vi "ZK_Main.vi"() -> ()   [LabVIEW 2018]
uses:
  C:/Users/rshang/Desktop/2020_APZK_LV360_Ricky/LabVIEWZOOKEPPER_V3/ClassLibrary_ZK.dll
  2020_APZK_LV360_Ricky/LabVIEWZOOKEPPER_V3/ClassLibrary_ZK.dll
  <vilib>/Utility/inputDevices.llb/keyboardAcquire.vi
  <vilib>/Utility/inputDevices.llb/closeKeyboard.vi
panel:
  out "Found?":bool=TRUE
  in  "Auto\n(Press keyboad\n A to stop)":bool
  in  "exe position":T1={"LU"={"x"=1456.0, "y"=98.0}, " RD"={"x"=1806.0, "y"=511.0}}
  out "Array":dbl[][](array[numeric])=[[0.0, 7.0, 4.0, 1.0, 7.0, 1.0, 7.0, 1.0], [5.0, 4.0, 6.0, 3.0, 7.0, 7.0, 1.0, 4.0], [3.0, 2.0, 4.0, 6.0, 1.0, 2.0, 7.0, 4.0], [5.0, 2.0, 6.0, 5.0, 4.0, 1.0, 4.0, 6.0], [3.0, 1.0, 2.0, 6.0, 5.0, 2.0, 4.0, 3.0], [4.0, 5.0, 1.0, 6.0, 1.0, 1.0, 7.0, 3.0], [6.0, 1.0, 2.0, 4.0, 4.0, 7.0, 3.0, 1.0], [6.0, 5.0, 2.0, 7.0, 3.0, 5.0, 3.0, 1.0]]
  out "Title":string="Zookeeper LabVIEW auto-player"
  out "Auto":bool
  in  "mouse setting":cluster{"X1":i32, "Y1":i32, "X2":i32, "Y2":i32}={"X1"=1479, "Y1"=217, "X2"=1733, "Y2"=457}
  in  "stop":bool
  out "Calibrated Matches 2":T2(array[cluster])=[[{"Position"={"x"=75.00092, "y"=255.0092}, "Angle"=0.0, "Scale"=1.0, "Score"=933.23773, "Bounding Box"=[{"x"=58.000923, "y"=238.0092}, {"x"=91.00092, "y"=238.0092}, {"x"=91.00092, "y"=271.00922}, {"x"=58.000923, "y"=271.00922}, {"x"=58.000923, "y"=238.0092}]}, {"Position"={"x"=279.0, "y"=323.0}, "Angle"=0.0, "Scale"=1.0, "Score"=932.08344, "Bounding Box"=[{"x"=262.0, "y"=306.0}, {"x"=295.0, "y"=306.0}, {"x"=295.0, "y"=339.0}, {"x"=262.0, "y"=339.0}, {"x"=262.0, "y"=306.0}]}, {"Position"={"x"=210.99873, "y"=119.0105}, "Angle"=0.0, "Scale"=1.0, "Score"=930.9997, "Bounding Box"=[{"x"=193.99873, "y"=102.0105}, {"x"=226.99873, "y"=102.0105}, {"x"=226.99873, "y"=135.0105}, {"x"=193.99873, "y"=135.0105}, {"x"=193.99873, "y"=102.0105}]}, {"Position"={"x"=176.99084, "y"=289.02286}, "Angle"=0.0, "Scale"=1.0, "Score"=925.0761, "Bounding Box"=[{"x"=159.99084, "y"=272.02286}, {"x"=192.99084, "y"=272.02286}, {"x"=192.99084, "y"=305.02286}, {"x"=159.99084, "y"=305.02286}, {"x"=159.99084, "y"=272.02286}]}, {"Position"={"x"=210.99141, "y"=288.9893}, "Angle"=0.0, "Scale"=1.0, "Score"=925.0041, "Bounding Box"=[{"x"=193.99141, "y"=271.9893}, {"x"=226.99141, "y"=271.9893}, {"x"=226.99141, "y"=304.9893}, {"x"=193.99141, "y"=304.9893}, {"x"=193.99141, "y"=271.9893}]}, {"Position"={"x"=142.99681, "y"=119.04378}, "Angle"=0.0, "Scale"=1.0, "Score"=920.4134, "Bounding Box"=[{"x"=125.99681, "y"=102.04378}, {"x"=158.99681, "y"=102.04378}, {"x"=158.99681, "y"=135.04378}, {"x"=125.99681, "y"=135.04378}, {"x"=125.99681, "y"=102.04378}]}, {"Position"={"x"=278.99835, "y"=119.04145}, "Angle"=0.0, "Scale"=1.0, "Score"=912.4555, "Bounding Box"=[{"x"=261.99835, "y"=102.04145}, {"x"=294.99835, "y"=102.04145}, {"x"=294.99835, "y"=135.04144}, {"x"=261.99835, "y"=135.04144}, {"x"=261.99835, "y"=102.04145}]}, {"Position"={"x"=245.00299, "y"=153.00949}, "Angle"=0.0, "Scale"=1.0, "Score"=905.00775, "Bounding Box"=[{"x"=228.00299, "y"=136.00949}, {"x"=261.003, "y"=136.00949}, {"x"=261.003, "y"=169.00949}, {"x"=228.00299, "y"=169.00949}, {"x"=228.00299, "y"=136.00949}]}, {"Position"={"x"=177.00247, "y"=186.99414}, "Angle"=0.0, "Scale"=1.0, "Score"=904.1407, "Bounding Box"=[{"x"=160.00247, "y"=169.99414}, {"x"=193.00247, "y"=169.99414}, {"x"=193.00247, "y"=202.99414}, {"x"=160.00247, "y"=202.99414}, {"x"=160.00247, "y"=169.99414}]}, {"Position"={"x"=210.99931, "y"=220.98695}, "Angle"=0.0, "Scale"=1.0, "Score"=901.1566, "Bounding Box"=[{"x"=193.99931, "y"=203.98695}, {"x"=226.99931, "y"=203.98695}, {"x"=226.99931, "y"=236.98695}, {"x"=193.99931, "y"=236.98695}, {"x"=193.99931, "y"=203.98695}]}, {"Position"={"x"=109.00134, "y"=289.00165}, "Angle"=0.0, "Scale"=1.0, "Score"=887.957, "Bounding Box"=[{"x"=92.00134, "y"=272.00165}, {"x"=125.00134, "y"=272.00165}, {"x"=125.00134, "y"=305.00165}, {"x"=92.00134, "y"=305.00165}, {"x"=92.00134, "y"=272.00165}]}, {"Position"={"x"=75.00068, "y"=323.03723}, "Angle"=0.0, "Scale"=1.0, "Score"=884.5231, "Bounding Box"=[{"x"=58.00068, "y"=306.03723}, {"x"=91.00068, "y"=306.03723}, {"x"=91.00068, "y"=339.03723}, {"x"=58.00068, "y"=339.03723}, {"x"=58.00068, "y"=306.03723}]}, {"Position"={"x"=273.11758, "y"=362.57874}, "Angle"=0.0, "Scale"=1.0, "Score"=841.5791, "Bounding Box"=[{"x"=256.11758, "y"=345.57874}, {"x"=289.11758, "y"=345.57874}, {"x"=289.11758, "y"=378.57874}, {"x"=256.11758, "y"=378.57874}, {"x"=256.11758, "y"=345.57874}]}], [{"Position"={"x"=107.986984, "y"=323.99716}, "Angle"=0.0, "Scale"=1.0, "Score"=931.8045, "Bounding Box"=[{"x"=92.986984, "y"=307.99716}, {"x"=121.986984, "y"=307.99716}, {"x"=121.986984, "y"=338.99716}, {"x"=92.986984, "y"=338.99716}, {"x"=92.986984, "y"=307.99716}]}, {"Position"={"x"=74.068016, "y"=221.99124}, "Angle"=0.0, "Scale"=1.0, "Score"=925.1344, "Bounding Box"=[{"x"=59.068016, "y"=205.99124}, {"x"=88.068016, "y"=205.99124}, {"x"=88.068016, "y"=236.99124}, {"x"=59.068016, "y"=236.99124}, {"x"=59.068016, "y"=205.99124}]}, {"Position"={"x"=210.09818, "y"=256.00165}, "Angle"=0.0, "Scale"=1.0, "Score"=920.25055, "Bounding Box"=[{"x"=195.09818, "y"=240.00165}, {"x"=224.09818, "y"=240.00165}, {"x"=224.09818, "y"=271.00165}, {"x"=195.09818, "y"=271.00165}, {"x"=195.09818, "y"=240.00165}]}, {"Position"={"x"=108.11167, "y"=256.0057}, "Angle"=0.0, "Scale"=1.0, "Score"=915.52545, "Bounding Box"=[{"x"=93.11167, "y"=240.0057}, {"x"=122.11167, "y"=240.0057}, {"x"=122.11167, "y"=271.0057}, {"x"=93.11167, "y"=271.0057}, {"x"=93.11167, "y"=240.0057}]}, {"Position"={"x"=209.99649, "y"=188.00977}, "Angle"=0.0, "Scale"=1.0, "Score"=910.0421, "Bounding Box"=[{"x"=194.99649, "y"=172.00977}, {"x"=223.99649, "y"=172.00977}, {"x"=223.99649, "y"=203.00977}, {"x"=194.99649, "y"=203.00977}, {"x"=194.99649, "y"=172.00977}]}, {"Position"={"x"=107.98176, "y"=357.98648}, "Angle"=0.0, "Scale"=1.0, "Score"=894.9287, "Bounding Box"=[{"x"=92.98176, "y"=341.98648}, {"x"=121.98176, "y"=341.98648}, {"x"=121.98176, "y"=372.98648}, {"x"=92.98176, "y"=372.98648}, {"x"=92.98176, "y"=341.98648}]}, {"Position"={"x"=74.02244, "y"=188.00812}, "Angle"=0.0, "Scale"=1.0, "Score"=888.29694, "Bounding Box"=[{"x"=59.022438, "y"=172.00812}, {"x"=88.02244, "y"=172.00812}, {"x"=88.02244, "y"=203.00812}, {"x"=59.022438, "y"=203.00812}, {"x"=59.022438, "y"=172.00812}]}, {"Position"={"x"=0.0, "y"=0.0}, "Angle"=0.0, "Scale"=0.0, "Score"=0.0, "Bounding Box"=[]}, {"Position"={"x"=0.0, "y"=0.0}, "Angle"=0.0, "Scale"=0.0, "Score"=0.0, "Bounding Box"=[]}, {"Position"={"x"=0.0, "y"=0.0}, "Angle"=0.0, "Scale"=0.0, "Score"=0.0, "Bounding Box"=[]}, {"Position"={"x"=0.0, "y"=0.0}, "Angle"=0.0, "Scale"=0.0, "Score"=0.0, "Bounding Box"=[]}, {"Position"={"x"=0.0, "y"=0.0}, "Angle"=0.0, "Scale"=0.0, "Score"=0.0, "Bounding Box"=[]}, {"Position"={"x"=0.0, "y"=0.0}, "Angle"=0.0, "Scale"=0.0, "Score"=0.0, "Bounding Box"=[]}], [{"Position"={"x"=277.90146, "y"=289.0273}, "Angle"=0.0, "Scale"=1.0, "Score"=926.91986, "Bounding Box"=[{"x"=261.90146, "y"=272.0273}, {"x"=292.90146, "y"=272.0273}, {"x"=292.90146, "y"=305.0273}, {"x"=261.90146, "y"=305.0273}, {"x"=261.90146, "y"=272.0273}]}, {"Position"={"x"=142.0333, "y"=153.05386}, "Angle"=0.0, "Scale"=1.0, "Score"=920.6298, "Bounding Box"=[{"x"=126.033295, "y"=136.05386}, {"x"=157.0333, "y"=136.05386}, {"x"=157.0333, "y"=169.05386}, {"x"=126.033295, "y"=169.05386}, {"x"=126.033295, "y"=136.05386}]}, {"Position"={"x"=176.00894, "y"=357.03848}, "Angle"=0.0, "Scale"=1.0, "Score"=920.4684, "Bounding Box"=[{"x"=160.00894, "y"=340.03848}, {"x"=191.00894, "y"=340.03848}, {"x"=191.00894, "y"=373.03848}, {"x"=160.00894, "y"=373.03848}, {"x"=160.00894, "y"=340.03848}]}, {"Position"={"x"=243.82567, "y"=357.03494}, "Angle"=0.0, "Scale"=1.0, "Score"=917.59546, "Bounding Box"=[{"x"=227.82567, "y"=340.03494}, {"x"=258.82568, "y"=340.03494}, {"x"=258.82568, "y"=373.03494}, {"x"=227.82567, "y"=373.03494}, {"x"=227.82567, "y"=340.03494}]}, {"Position"={"x"=40.012535, "y"=187.0207}, "Angle"=0.0, "Scale"=1.0, "Score"=903.5547, "Bounding Box"=[{"x"=24.012535, "y"=170.0207}, {"x"=55.012535, "y"=170.0207}, {"x"=55.012535, "y"=203.0207}, {"x"=24.012535, "y"=203.0207}, {"x"=24.012535, "y"=170.0207}]}, {"Position"={"x"=40.08889, "y"=255.02586}, "Angle"=0.0, "Scale"=1.0, "Score"=899.9424, "Bounding Box"=[{"x"=24.08889, "y"=238.02586}, {"x"=55.08889, "y"=238.02586}, {"x"=55.08889, "y"=271.02588}, {"x"=24.08889, "y"=271.02588}, {"x"=24.08889, "y"=238.02586}]}, {"Position"={"x"=244.2408, "y"=323.06232}, "Angle"=0.0, "Scale"=1.0, "Score"=899.3051, "Bounding Box"=[{"x"=228.2408, "y"=306.06232}, {"x"=259.24078, "y"=306.06232}, {"x"=259.24078, "y"=339.06232}, {"x"=228.2408, "y"=339.06232}, {"x"=228.2408, "y"=306.06232}]}, {"Position"={"x"=277.75967, "y"=255.03061}, "Angle"=0.0, "Scale"=1.0, "Score"=894.2649, "Bounding Box"=[{"x"=261.75967, "y"=238.03061}, {"x"=292.75967, "y"=238.03061}, {"x"=292.75967, "y"=271.0306}, {"x"=261.75967, "y"=271.0306}, {"x"=261.75967, "y"=238.03061}]}, {"Position"={"x"=0.0, "y"=0.0}, "Angle"=0.0, "Scale"=0.0, "Score"=0.0, "Bounding Box"=[]}, {"Position"={"x"=0.0, "y"=0.0}, "Angle"=0.0, "Scale"=0.0, "Score"=0.0, "Bounding Box"=[]}, {"Position"={"x"=0.0, "y"=0.0}, "Angle"=0.0, "Scale"=0.0, "Score"=0.0, "Bounding Box"=[]}, {"Position"={"x"=0.0, "y"=0.0}, "Angle"=0.0, "Scale"=0.0, "Score"=0.0, "Bounding Box"=[]}, {"Position"={"x"=0.0, "y"=0.0}, "Angle"=0.0, "Scale"=0.0, "Score"=0.0, "Bounding Box"=[]}], [{"Position"={"x"=245.00069, "y"=254.18097}, "Angle"=0.0, "Scale"=1.0, "Score"=954.2915, "Bounding Box"=[{"x"=230.00069, "y"=238.18097}, {"x"=260.00067, "y"=238.18097}, {"x"=260.00067, "y"=269.18097}, {"x"=230.00069, "y"=269.18097}, {"x"=230.00069, "y"=238.18097}]}, {"Position"={"x"=279.13513, "y"=152.48029}, "Angle"=0.0, "Scale"=1.0, "Score"=940.6921, "Bounding Box"=[{"x"=264.13513, "y"=136.48029}, {"x"=294.13513, "y"=136.48029}, {"x"=294.13513, "y"=167.48029}, {"x"=264.13513, "y"=167.48029}, {"x"=264.13513, "y"=136.48029}]}, {"Position"={"x"=109.067566, "y"=186.16963}, "Angle"=0.0, "Scale"=1.0, "Score"=938.7648, "Bounding Box"=[{"x"=94.067566, "y"=170.16963}, {"x"=124.067566, "y"=170.16963}, {"x"=124.067566, "y"=201.16963}, {"x"=94.067566, "y"=201.16963}, {"x"=94.067566, "y"=170.16963}]}, {"Position"={"x"=177.16257, "y"=322.33588}, "Angle"=0.0, "Scale"=1.0, "Score"=933.9336, "Bounding Box"=[{"x"=162.16257, "y"=306.33588}, {"x"=192.16257, "y"=306.33588}, {"x"=192.16257, "y"=337.33588}, {"x"=162.16257, "y"=337.33588}, {"x"=162.16257, "y"=306.33588}]}, {"Position"={"x"=75.14856, "y"=152.44539}, "Angle"=0.0, "Scale"=1.0, "Score"=927.445, "Bounding Box"=[{"x"=60.14856, "y"=136.44539}, {"x"=90.14856, "y"=136.44539}, {"x"=90.14856, "y"=167.44539}, {"x"=60.14856, "y"=167.44539}, {"x"=60.14856, "y"=136.44539}]}, {"Position"={"x"=108.93101, "y"=118.46414}, "Angle"=0.0, "Scale"=1.0, "Score"=922.298, "Bounding Box"=[{"x"=93.93101, "y"=102.46414}, {"x"=123.93101, "y"=102.46414}, {"x"=123.93101, "y"=133.46414}, {"x"=93.93101, "y"=133.46414}, {"x"=93.93101, "y"=102.46414}]}, {"Position"={"x"=143.0, "y"=323.0}, "Angle"=0.0, "Scale"=1.0, "Score"=915.732, "Bounding Box"=[{"x"=128.0, "y"=307.0}, {"x"=158.0, "y"=307.0}, {"x"=158.0, "y"=338.0}, {"x"=128.0, "y"=338.0}, {"x"=128.0, "y"=307.0}]}, {"Position"={"x"=41.060474, "y"=288.27094}, "Angle"=0.0, "Scale"=1.0, "Score"=914.88336, "Bounding Box"=[{"x"=26.060474, "y"=272.27094}, {"x"=56.060474, "y"=272.27094}, {"x"=56.060474, "y"=303.27094}, {"x"=26.060474, "y"=303.27094}, {"x"=26.060474, "y"=272.27094}]}, {"Position"={"x"=244.9803, "y"=220.15024}, "Angle"=0.0, "Scale"=1.0, "Score"=913.309, "Bounding Box"=[{"x"=229.9803, "y"=204.15024}, {"x"=259.9803, "y"=204.15024}, {"x"=259.9803, "y"=235.15024}, {"x"=229.9803, "y"=235.15024}, {"x"=229.9803, "y"=204.15024}]}, {"Position"={"x"=279.1057, "y"=185.95796}, "Angle"=0.0, "Scale"=1.0, "Score"=905.5621, "Bounding Box"=[{"x"=264.1057, "y"=169.95796}, {"x"=294.1057, "y"=169.95796}, {"x"=294.1057, "y"=200.95796}, {"x"=264.1057, "y"=200.95796}, {"x"=264.1057, "y"=169.95796}]}, {"Position"={"x"=176.76869, "y"=220.71819}, "Angle"=0.0, "Scale"=1.0, "Score"=901.4693, "Bounding Box"=[{"x"=161.76869, "y"=204.71819}, {"x"=191.76869, "y"=204.71819}, {"x"=191.76869, "y"=235.71819}, {"x"=161.76869, "y"=235.71819}, {"x"=161.76869, "y"=204.71819}]}, {"Position"={"x"=0.0, "y"=0.0}, "Angle"=0.0, "Scale"=0.0, "Score"=0.0, "Bounding Box"=[]}, {"Position"={"x"=0.0, "y"=0.0}, "Angle"=0.0, "Scale"=0.0, "Score"=0.0, "Bounding Box"=[]}], [{"Position"={"x"=74.0, "y"=355.0}, "Angle"=0.0, "Scale"=1.0, "Score"=919.12885, "Bounding Box"=[{"x"=58.0, "y"=339.0}, {"x"=90.0, "y"=339.0}, {"x"=90.0, "y"=371.0}, {"x"=58.0, "y"=371.0}, {"x"=58.0, "y"=339.0}]}, {"Position"={"x"=73.991066, "y"=287.9914}, "Angle"=0.0, "Scale"=1.0, "Score"=878.5044, "Bounding Box"=[{"x"=57.991066, "y"=271.9914}, {"x"=89.991066, "y"=271.9914}, {"x"=89.991066, "y"=303.9914}, {"x"=57.991066, "y"=303.9914}, {"x"=57.991066, "y"=271.9914}]}, {"Position"={"x"=27.626839, "y"=210.72752}, "Angle"=0.0, "Scale"=1.0, "Score"=863.36957, "Bounding Box"=[{"x"=11.626839, "y"=194.72752}, {"x"=43.62684, "y"=194.72752}, {"x"=43.62684, "y"=226.72752}, {"x"=11.626839, "y"=226.72752}, {"x"=11.626839, "y"=194.72752}]}, {"Position"={"x"=209.92537, "y"=356.0048}, "Angle"=0.0, "Scale"=1.0, "Score"=856.84375, "Bounding Box"=[{"x"=193.92537, "y"=340.0048}, {"x"=225.92537, "y"=340.0048}, {"x"=225.92537, "y"=372.0048}, {"x"=193.92537, "y"=372.0048}, {"x"=193.92537, "y"=340.0048}]}, {"Position"={"x"=175.98193, "y"=253.99306}, "Angle"=0.0, "Scale"=1.0, "Score"=848.5472, "Bounding Box"=[{"x"=159.98193, "y"=237.99306}, {"x"=191.98193, "y"=237.99306}, {"x"=191.98193, "y"=269.99304}, {"x"=159.98193, "y"=269.99304}, {"x"=159.98193, "y"=237.99306}]}, {"Position"={"x"=141.95236, "y"=220.00485}, "Angle"=0.0, "Scale"=1.0, "Score"=844.96405, "Bounding Box"=[{"x"=125.95236, "y"=204.00485}, {"x"=157.95236, "y"=204.00485}, {"x"=157.95236, "y"=236.00485}, {"x"=125.95236, "y"=236.00485}, {"x"=125.95236, "y"=204.00485}]}, {"Position"={"x"=27.773817, "y"=140.42613}, "Angle"=0.0, "Scale"=1.0, "Score"=830.67377, "Bounding Box"=[{"x"=11.773817, "y"=124.42613}, {"x"=43.77382, "y"=124.42613}, {"x"=43.77382, "y"=156.42613}, {"x"=11.773817, "y"=156.42613}, {"x"=11.773817, "y"=124.42613}]}, {"Position"={"x"=191.0, "y"=374.0}, "Angle"=0.0, "Scale"=1.0, "Score"=814.83405, "Bounding Box"=[{"x"=175.0, "y"=358.0}, {"x"=207.0, "y"=358.0}, {"x"=207.0, "y"=390.0}, {"x"=175.0, "y"=390.0}, {"x"=175.0, "y"=358.0}]}, {"Position"={"x"=0.0, "y"=0.0}, "Angle"=0.0, "Scale"=0.0, "Score"=0.0, "Bounding Box"=[]}, {"Position"={"x"=0.0, "y"=0.0}, "Angle"=0.0, "Scale"=0.0, "Score"=0.0, "Bounding Box"=[]}, {"Position"={"x"=0.0, "y"=0.0}, "Angle"=0.0, "Scale"=0.0, "Score"=0.0, "Bounding Box"=[]}, {"Position"={"x"=0.0, "y"=0.0}, "Angle"=0.0, "Scale"=0.0, "Score"=0.0, "Bounding Box"=[]}, {"Position"={"x"=0.0, "y"=0.0}, "Angle"=0.0, "Scale"=0.0, "Score"=0.0, "Bounding Box"=[]}], [{"Position"={"x"=108.99241, "y"=153.01335}, "Angle"=0.0, "Scale"=1.0, "Score"=950.8153, "Bounding Box"=[{"x"=92.99241, "y"=136.01335}, {"x"=123.99241, "y"=136.01335}, {"x"=123.99241, "y"=170.01335}, {"x"=92.99241, "y"=170.01335}, {"x"=92.99241, "y"=136.01335}]}, {"Position"={"x"=109.00232, "y"=221.00328}, "Angle"=0.0, "Scale"=1.0, "Score"=950.37427, "Bounding Box"=[{"x"=93.00232, "y"=204.00328}, {"x"=124.00232, "y"=204.00328}, {"x"=124.00232, "y"=238.00328}, {"x"=93.00232, "y"=238.00328}, {"x"=93.00232, "y"=204.00328}]}, {"Position"={"x"=142.97572, "y"=187.00519}, "Angle"=0.0, "Scale"=1.0, "Score"=949.1306, "Bounding Box"=[{"x"=126.97572, "y"=170.00519}, {"x"=157.97572, "y"=170.00519}, {"x"=157.97572, "y"=204.00519}, {"x"=126.97572, "y"=204.00519}, {"x"=126.97572, "y"=170.00519}]}, {"Position"={"x"=278.84097, "y"=220.9837}, "Angle"=0.0, "Scale"=1.0, "Score"=935.6025, "Bounding Box"=[{"x"=262.84097, "y"=203.9837}, {"x"=293.84097, "y"=203.9837}, {"x"=293.84097, "y"=237.9837}, {"x"=262.84097, "y"=237.9837}, {"x"=262.84097, "y"=203.9837}]}, {"Position"={"x"=143.0, "y"=289.0}, "Angle"=0.0, "Scale"=1.0, "Score"=926.99817, "Bounding Box"=[{"x"=127.0, "y"=272.0}, {"x"=158.0, "y"=272.0}, {"x"=158.0, "y"=306.0}, {"x"=127.0, "y"=306.0}, {"x"=127.0, "y"=272.0}]}, {"Position"={"x"=142.79024, "y"=255.01186}, "Angle"=0.0, "Scale"=1.0, "Score"=919.38403, "Bounding Box"=[{"x"=126.79024, "y"=238.01186}, {"x"=157.79024, "y"=238.01186}, {"x"=157.79024, "y"=272.01184}, {"x"=126.79024, "y"=272.01184}, {"x"=126.79024, "y"=238.01186}]}, {"Position"={"x"=41.008556, "y"=323.00058}, "Angle"=0.0, "Scale"=1.0, "Score"=916.4105, "Bounding Box"=[{"x"=25.008556, "y"=306.00058}, {"x"=56.008556, "y"=306.00058}, {"x"=56.008556, "y"=340.00058}, {"x"=25.008556, "y"=340.00058}, {"x"=25.008556, "y"=306.00058}]}, {"Position"={"x"=40.85029, "y"=356.99994}, "Angle"=0.0, "Scale"=1.0, "Score"=915.2918, "Bounding Box"=[{"x"=24.850288, "y"=339.99994}, {"x"=55.85029, "y"=339.99994}, {"x"=55.85029, "y"=373.99994}, {"x"=24.850288, "y"=373.99994}, {"x"=24.850288, "y"=339.99994}]}, {"Position"={"x"=0.0, "y"=0.0}, "Angle"=0.0, "Scale"=0.0, "Score"=0.0, "Bounding Box"=[]}, {"Position"={"x"=0.0, "y"=0.0}, "Angle"=0.0, "Scale"=0.0, "Score"=0.0, "Bounding Box"=[]}, {"Position"={"x"=0.0, "y"=0.0}, "Angle"=0.0, "Scale"=0.0, "Score"=0.0, "Bounding Box"=[]}, {"Position"={"x"=0.0, "y"=0.0}, "Angle"=0.0, "Scale"=0.0, "Score"=0.0, "Bounding Box"=[]}, {"Position"={"x"=0.0, "y"=0.0}, "Angle"=0.0, "Scale"=0.0, "Score"=0.0, "Bounding Box"=[]}], [{"Position"={"x"=142.00067, "y"=357.00705}, "Angle"=0.0, "Scale"=1.0, "Score"=918.7663, "Bounding Box"=[{"x"=125.00067, "y"=340.00705}, {"x"=159.00067, "y"=340.00705}, {"x"=159.00067, "y"=374.00705}, {"x"=125.00067, "y"=374.00705}, {"x"=125.00067, "y"=340.00705}]}, {"Position"={"x"=209.99313, "y"=153.00714}, "Angle"=0.0, "Scale"=1.0, "Score"=915.01294, "Bounding Box"=[{"x"=192.99313, "y"=136.00714}, {"x"=226.99313, "y"=136.00714}, {"x"=226.99313, "y"=170.00714}, {"x"=192.99313, "y"=170.00714}, {"x"=192.99313, "y"=136.00714}]}, {"Position"={"x"=175.99594, "y"=119.00965}, "Angle"=0.0, "Scale"=1.0, "Score"=909.40247, "Bounding Box"=[{"x"=158.99594, "y"=102.00965}, {"x"=192.99594, "y"=102.00965}, {"x"=192.99594, "y"=136.00964}, {"x"=158.99594, "y"=136.00964}, {"x"=158.99594, "y"=102.00965}]}, {"Position"={"x"=209.96707, "y"=323.00375}, "Angle"=0.0, "Scale"=1.0, "Score"=900.32886, "Bounding Box"=[{"x"=192.96707, "y"=306.00375}, {"x"=226.96707, "y"=306.00375}, {"x"=226.96707, "y"=340.00375}, {"x"=192.96707, "y"=340.00375}, {"x"=192.96707, "y"=306.00375}]}, {"Position"={"x"=175.96883, "y"=153.0146}, "Angle"=0.0, "Scale"=1.0, "Score"=894.0803, "Bounding Box"=[{"x"=158.96883, "y"=136.0146}, {"x"=192.96883, "y"=136.0146}, {"x"=192.96883, "y"=170.0146}, {"x"=158.96883, "y"=170.0146}, {"x"=158.96883, "y"=136.0146}]}, {"Position"={"x"=243.96931, "y"=289.00467}, "Angle"=0.0, "Scale"=1.0, "Score"=893.323, "Bounding Box"=[{"x"=226.96931, "y"=272.00467}, {"x"=260.9693, "y"=272.00467}, {"x"=260.9693, "y"=306.00467}, {"x"=226.96931, "y"=306.00467}, {"x"=226.96931, "y"=272.00467}]}, {"Position"={"x"=73.975296, "y"=119.0135}, "Angle"=0.0, "Scale"=1.0, "Score"=889.3833, "Bounding Box"=[{"x"=56.975296, "y"=102.0135}, {"x"=90.975296, "y"=102.0135}, {"x"=90.975296, "y"=136.01349}, {"x"=56.975296, "y"=136.01349}, {"x"=56.975296, "y"=102.0135}]}, {"Position"={"x"=243.99707, "y"=187.014}, "Angle"=0.0, "Scale"=1.0, "Score"=888.0418, "Bounding Box"=[{"x"=226.99707, "y"=170.014}, {"x"=260.99707, "y"=170.014}, {"x"=260.99707, "y"=204.014}, {"x"=226.99707, "y"=204.014}, {"x"=226.99707, "y"=170.014}]}, {"Position"={"x"=243.99458, "y"=119.01848}, "Angle"=0.0, "Scale"=1.0, "Score"=872.4473, "Bounding Box"=[{"x"=226.99458, "y"=102.01848}, {"x"=260.99457, "y"=102.01848}, {"x"=260.99457, "y"=136.01848}, {"x"=226.99458, "y"=136.01848}, {"x"=226.99458, "y"=102.01848}]}, {"Position"={"x"=0.0, "y"=0.0}, "Angle"=0.0, "Scale"=0.0, "Score"=0.0, "Bounding Box"=[]}, {"Position"={"x"=0.0, "y"=0.0}, "Angle"=0.0, "Scale"=0.0, "Score"=0.0, "Bounding Box"=[]}, {"Position"={"x"=0.0, "y"=0.0}, "Angle"=0.0, "Scale"=0.0, "Score"=0.0, "Bounding Box"=[]}, {"Position"={"x"=0.0, "y"=0.0}, "Angle"=0.0, "Scale"=0.0, "Score"=0.0, "Bounding Box"=[]}]]
  out "mouseposition":string="412@228"
  out "Image Out":T3(plugin-control)
  # "Animal"
  # "Ricky_version 3"
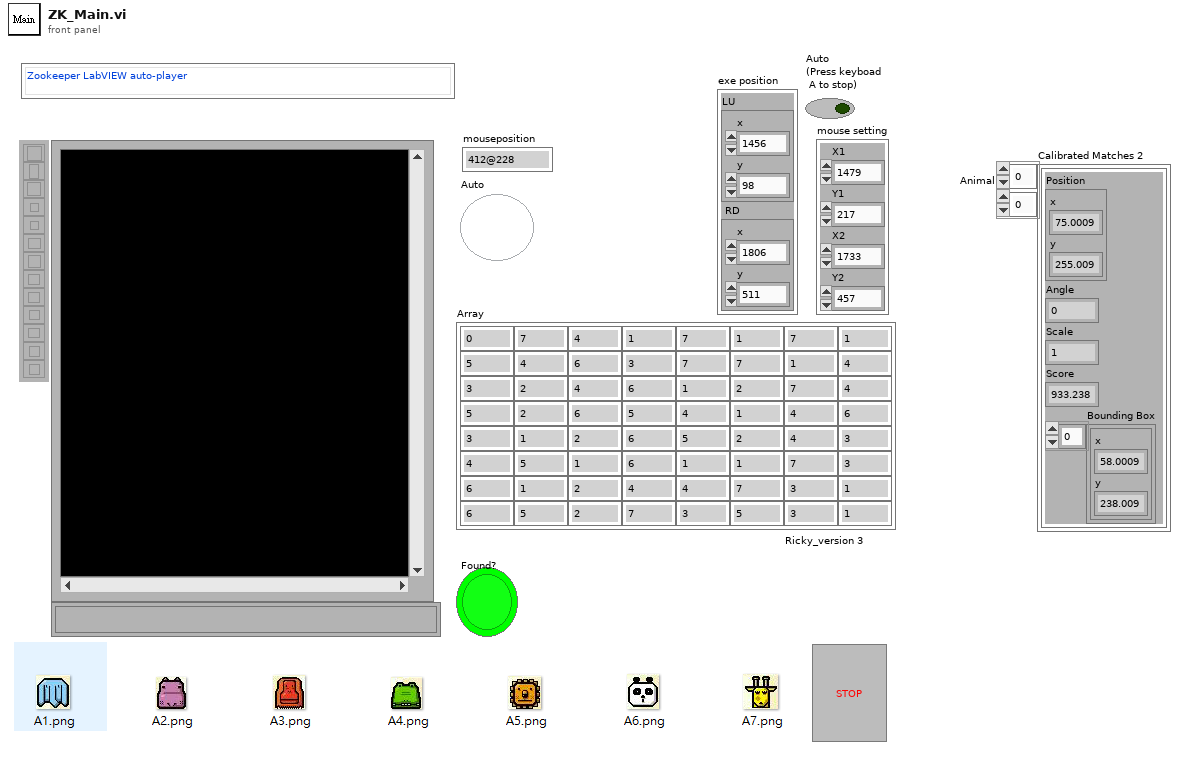
[diagram p1: front panel]
types:
  T1 = cluster{"LU":cluster{"x":sgl, "y":sgl}, " RD":cluster{"x":sgl, "y":sgl}}
  T2 = cluster{"Position":cluster{"x":sgl, "y":sgl}, "Angle":sgl, "Scale":sgl, "Score":sgl, "Bounding Box":cluster{"x":sgl, "y":sgl}[]}[][]
  T3 = typedef "IMAQ Image.ctl" = refnum<image>
  T4 = enum16{"0", "1", "2", "3", "4", "5", "6", "7", "8", "9", "A", "B", "C", "D", "E", "F", "G", "H", "I", "J", "K", "L", "M", "N", "O", "P", "Q", "R", "S", "T", "U", "V", "W", "X", "Y", "Z", "F1", "F2", "F3", "F4", "F5", "F6", "F7", "F8", "F9", "F10", "F11", "F12", "F13", "F14", "F15", "ADD", "BACK", "BACKSLASH", "CAPITAL", "COMMA", "DECIMAL", "DELETE", "DIVIDE", "DOWN", "END", "EQUALS", "ESCAPE", "GRAVE (`)", "HOME", "INSERT", "LBRACKET", "LCONTROL", "LEFT", "L ALT", "LSHIFT", "LWIN", "MINUS", "MULTIPLY", "NEXT", "NUMLOCK", "NUMPAD_0", "NUMPAD_1", "NUMPAD_2", "NUMPAD_3", "NUMPAD_4", "NUMPAD_5", "NUMPAD_6", "NUMPAD_7", "NUMPAD_8", "NUMPAD_9", "PAUSE", "PERIOD", "PRIOR (PG UP)", "RBRACKET", "RCONTROL", "RETURN", "RIGHT", "R ALT", "RSHIFT", "RWIN", "SCROLL", "SEMICOLON", "SLASH", "SPACE", "SUBTRACT", "TAB", "UP", "ENTER (num pad)", "' (quote)"}
  T5 = enum16{"0", "1", "2", "3", "4", "5", "6", "7", "8", "9", "A", "B", "C", "D", "E", "F", "G", "H", "I", "J", "K", "L", "M", "N", "O", "P", "Q", "R", "S", "T", "U", "V", "W", "X", "Y", "Z", "F1", "F2", "F3", "F4", "F5", "F6", "F7", "F8", "F9", "F10", "F11", "F12", "F13", "F14", "F15", "ADD", "BACK", "BACKSLASH", "CAPITAL", "COMMA", "DECIMAL", "DELETE", "DIVIDE", "DOWN", "END", "EQUALS", "ESCAPE", "GRAVE (`)", "HOME", "INSERT", "LBRACKET", "LCONTROL", "LEFT", "L ALT", "LSHIFT", "LWIN", "MINUS", "MULTIPLY", "NEXT", "NUMLOCK", "NUMPAD_0", "NUMPAD_1", "NUMPAD_2", "NUMPAD_3", "NUMPAD_4", "NUMPAD_5", "NUMPAD_6", "NUMPAD_7", "NUMPAD_8", "NUMPAD_9", "PAUSE", "PERIOD", "PRIOR (PG UP)", "RBRACKET", "RCONTROL", "RETURN", "RIGHT", "R ALT", "RSHIFT", "RWIN", "SCROLL", "SEMICOLON", "SLASH", "SPACE", "SUBTRACT", "TAB", "UP", "ENTER (num pad)", "' (quote)"}[]
  T6 = cluster{"A_Row":i32, "A_Col":i32, "B_Row":i32, "B_Col":i32}
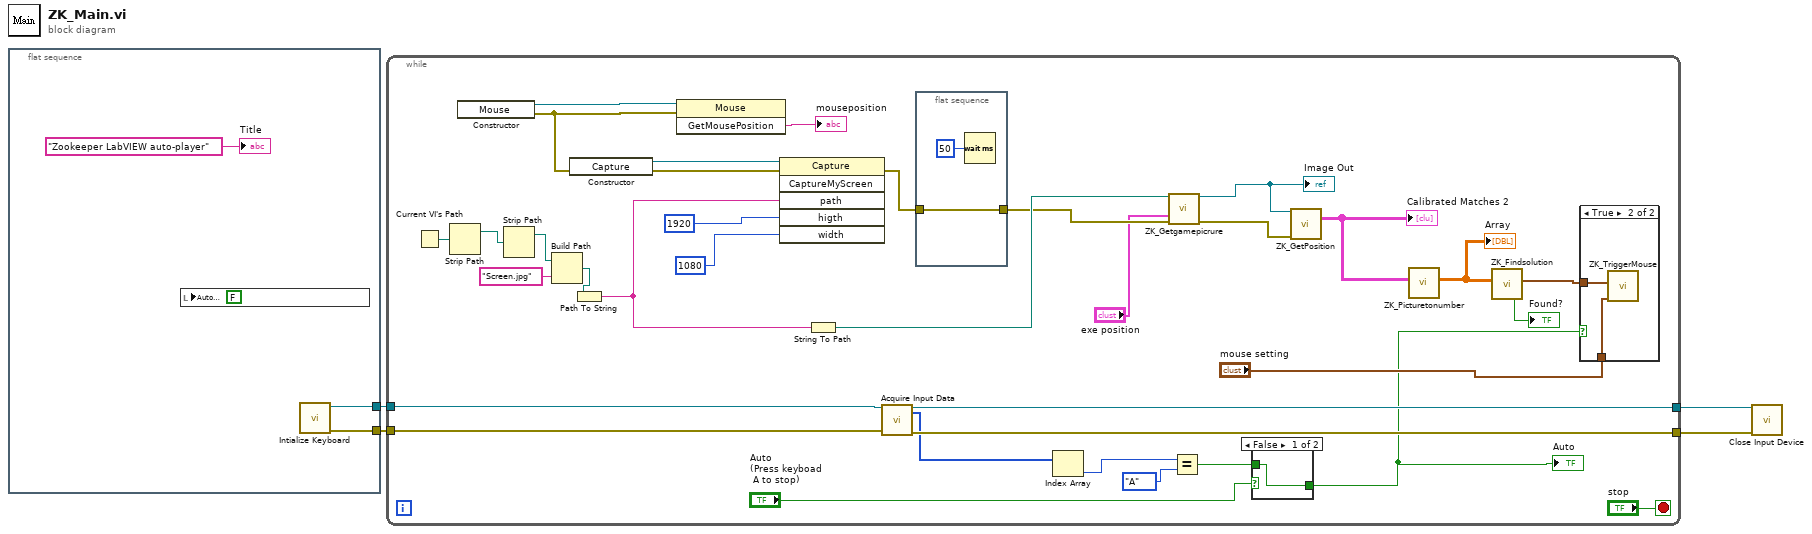
[diagram p0: block diagram]
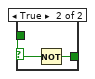
[diagram p2: hidden frame]
diagram:
  n1 = flat-sequence {
    tunnel: [w8] -> w4
    tunnel: [w7] -> w3
    frame #0 {
      n2 = local write "Auto\n(Press keyboad\n A to stop)"(FALSE ("Auto")) -> ()
      n3 = call <vilib>:"Intialize Keyboard.vi"() -> ("error out"=w7:errorcluster, "device ID"=w8:refnum<k1>)  [unwired: 10 in]
      "Title" <- "Zookeeper LabVIEW auto-player" ("Title")
    }
  }
  n4 = while {
    tunnel: w4 -> [w28]
    tunnel: w3 -> [w27]
    tunnel: [w26] -> w2
    tunnel: [w25] -> w1
    stop <- "stop" stop-if-true
    n5 = Current VI's Path() -> (path=w14:path)
    n6 = Strip Path(path=w14) -> (stripped path=w13:path)  [unwired: 1 out]
    n7 = constructor class="Mouse"() -> (reference out=w29:refnum<k24>, error out=w19:errorcluster)  [unwired: 3 in, 1 out]
    n8 = Strip Path(path=w13) -> (stripped path=w12:path)  [unwired: 1 out]
    n9 = Build Path(base path=w12, name or relative path="Screen.jpg") -> (appended path=w10:path)
    n10 = constructor class="Capture"(error in=w19) -> (reference out=w43:refnum<k24>, error out=w40:errorcluster)  [unwired: 2 in, 1 out]
    n11 = Path To String(path=w10) -> (string=w9:string)
    n12 = invoke class="Mouse" method="GetMousePosition"(reference=w29, error in=w19) -> ("GetMousePosition"=→"mouseposition":string)  [unwired: 1 in, 2 out]
    n13 = invoke class="Capture" method="CaptureMyScreen"(reference=w43, error in=w40, "path"=w9, "higth"=1920, "width"=1080 ("higth")) -> (error out=w37:errorcluster)  [unwired: 1 in, 5 out]
    n14 = String To Path(string=w9) -> (path=w39:path)
    n15 = call-poly <vilib>:"Acquire Input Data.vi"("device ID"=w28, "error in (no error)"=w27) -> ("device ID"=w26:refnum<k1>, "keys pressed"=w24:T5, "error out"=w25:errorcluster)  [unwired: 15 in]
    n16 = flat-sequence {
      tunnel: [w50] -> w38
      tunnel: w37 -> [w50]
      frame #0 {
        n17 = Wait (ms)(milliseconds to wait=u32 50) -> ()  [unwired: 1 out]
      }
    }
    n18 = Index Array(array=w24) -> (element=w23:T4)  [unwired: 1 in]
    n19 = call "ZK_Getgamepicrure.vi"("File Path"=w39, "Cluster 2"="exe position", "error in"=w38) -> ("Image Out"=w36:T3, "error out"=w20:errorcluster)  [unwired: 10 in, 1 out]
    "Image Out" <- w36
    n20 = Equal?(x=w23, y=T4."A") -> (x = y?=w18:bool)
    n21 = case shown="False" "Auto\n(Press keyboad\n A to stop)" {
      tunnel: w18 -> [w44 w46]
      tunnel: [w44 w45] -> w17
      frame False {
      }
      frame True {
        n22 = Not(x=w46) -> (.not. x?=w45:bool)
      }
    }
    "Auto" <- w17
    n23 = call "ZK_GetPosition.vi"("Image Out 2"=w36, "error in"=w20) -> ("Calibrated Matches 2"=w35:T2)  [unwired: 12 in, 1 out]
    "Calibrated Matches 2" <- w35
    n24 = call "ZK_Picturetonumber.vi"("Calibrated Matches 3"=w35) -> ("Array"=w34:dbl[][])  [unwired: 10 in]
    "Array" <- w34
    n25 = call "ZK_Findsolution.vi"("Array"=w34) -> ("f"=→"Found?":bool, "Result"=w33:T6)  [unwired: 9 in]
    n26 = case shown="True" w17 {
      tunnel: w33 -> [_ w48]
      tunnel: "mouse setting" -> [_ w47]
      frame False {
      }
      frame True {
        n27 = call "ZK_TriggerMouse.vi"("Cluster 3"=w47, "Result"=w48) -> ()  [unwired: 10 in]
      }
    }
  }
  n28 = call-poly <vilib>:"Close Input Device.vi"("error in (no error)"=w1, "device ID"=w2) -> ()  [unwired: 8 in, 1 out]
